vi "Read Wfm Data.vi"(8 "error in (no error)":errorcluster, 11 "Async State Vars in":T1) -> (0 "error out":errorcluster, 3 "Async State Vars out":T1, 4 "Wfm timed out?":bool)   [LabVIEW 2015, in "Waveform-Processing-Custom-Device Engine.lvlib"]
uses:
  Waveform-Processing-Custom-Device Engine.lvlib
  <vilib>/NI Veristand/Custom Device Waveform API/NI_VS Custom Device Waveform API.lvlib
  <vilib>/NI Veristand/Custom Device Waveform API/Single Waveform Read (DBL)/NI VeriStand - Read Single Waveform (DBL).vi
  <vilib>/NI Veristand/Custom Device Waveform API/Single Waveform Read (DBL)/Single Waveform Read (DBL).lvclass
  Built/Waveform-Processing-Custom-Device/c/Waveform-Processing-Custom-Device Engine Pharlap.llb/Circular Buffer(2D DBL).vi
  Built/Waveform-Processing-Custom-Device/c/Waveform-Processing-Custom-Device Engine Pharlap.llb/Circular Buffer.lvlib
  Built/Waveform-Processing-Custom-Device/c/Waveform-Processing-Custom-Device Engine Pharlap.llb/Circular Buffer Operations.ctl
  Types/Async FIFOs.ctl
  Types/Async State Vars.ctl
  <vilib>/NI Veristand/Custom Device Waveform API/Single Waveform Write (DBL)/Single Waveform Write (DBL).lvclass
  <vilib>/NI Veristand/Custom Device API/Waveform Data Reference.ctl
  <vilib>/NI VeriStand/Custom Device API/Custom Device API.lvlib
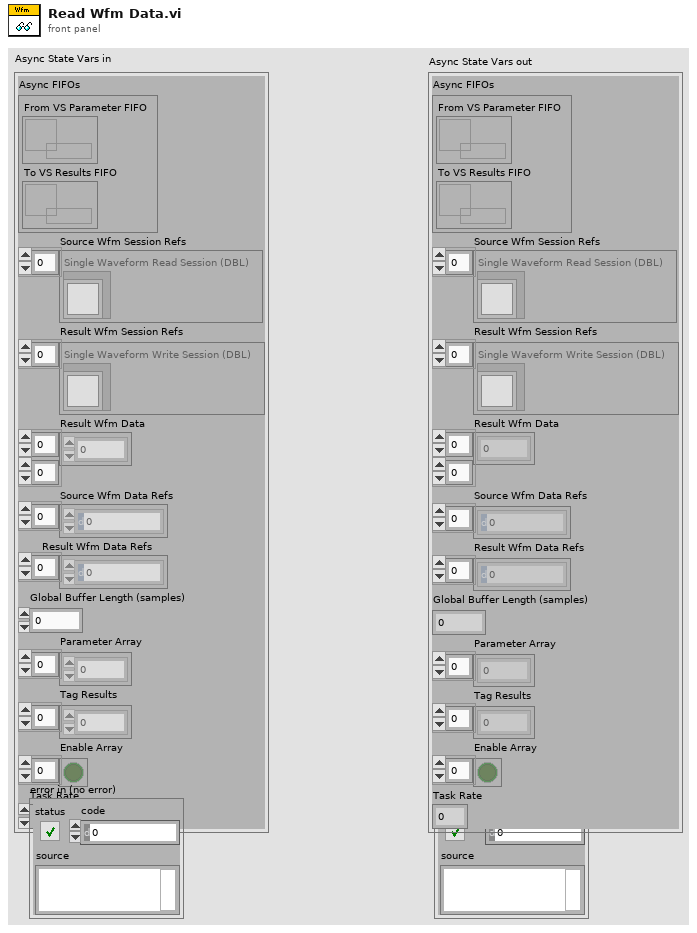
[diagram p1: front panel]
types:
  T1 = typedef "Waveform-Processing-Custom-Device Engine.lvlib/Async State Vars.ctl" = cluster{"Async FIFOs":T2, "Source Wfm Session Refs":refnum<class "Single Waveform Read (DBL).lvclass">[], "Result Wfm Session Refs":refnum<class "Single Waveform Write (DBL).lvclass">[], "Result Wfm Data":dbl[][], "Source Wfm Data Refs":T3[], "Result Wfm Data Refs":T3[], "Global Buffer Length (samples)":dbl, "Parameter Array":dbl[], "Tag Results":dbl[], "Enable Array":bool[], "Task Rate":dbl}
  T2 = typedef "Waveform-Processing-Custom-Device Engine.lvlib/Async FIFOs.ctl" = cluster{"From VS Parameter FIFO":refnum<k33>, "To VS Results FIFO":refnum<k33>}
  T3 = typedef "Custom Device API.lvlib/Waveform Data Reference.ctl" = i32
  T4 = typedef "Circular Buffer.lvlib/Circular Buffer Operations.ctl" = enum16{"Initialize", "Get Backlog", "Write", "Read (continuous)", "Read (most recent)"}
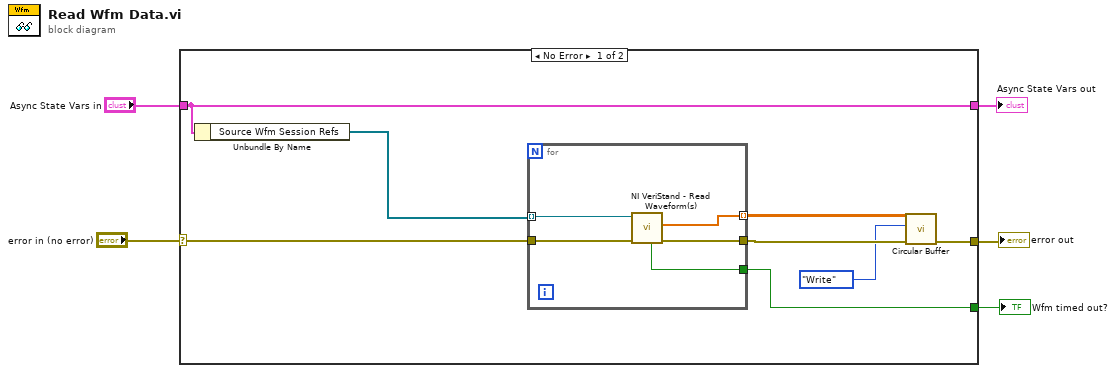
[diagram p0: block diagram]
diagram:
  n1 = case shown="No Error" "error in (no error)" {
    selector: "error in (no error)" -> [w8 w19]
    tunnel: [w9 w19] -> w5
    tunnel: "Async State Vars in" -> [w7 w20]
    tunnel: [w7 w20] -> w2
    tunnel: [w6 _] -> w1
    frame No Error {
      n2 = Unbundle By Name(w7) -> ("Source Wfm Session Refs"=w13:refnum<class "Single Waveform Read (DBL).lvclass">[])
      n3 = for {
        tunnel: w8 -> [w18]
        tunnel: [w17] -> w12
        tunnel: [w16] -> w10 mode=indexing
        tunnel: [w15] -> w6
        tunnel: w13 -> [w14] mode=indexing
        n4 = call-poly <vilib>:"NI VeriStand - Read Waveform(s).vi"("error in (no error)"=w18, "Single Waveform Read Session (DBL) in"=w14) -> ("error out"=w17:errorcluster, "Data"=w16:dbl[], "timed out?"=w15:bool)  [unwired: 5 in, 2 out]
      }
      n5 = call-poly <userlib>:"Circular Buffer.vi"("error in (no error)"=w12, "Operation"=Circular_Buffer_Operations."Write", "Data In"=w10) -> ("error out"=w9:errorcluster)  [unwired: 5 in, 3 out]
    }
    frame Error {
    }
  }
  "error out" <- w5
  "Wfm timed out?" <- w1
  "Async State Vars out" <- w2
